vi "Site List to Site Numbers.vi"(0 "Site List":string) -> (4 "Site Numbers":i32[](array[numeric]), 6 "Sites":string[](array[string]))   [LabVIEW 2020]
uses:
  <vilib>/Utility/error.llb/whitespace.ctl
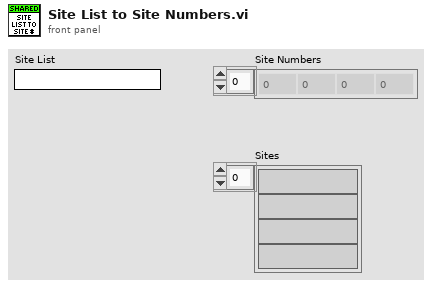
[diagram p1: front panel]
types:
  T1 = typedef "whitespace.ctl" = u16
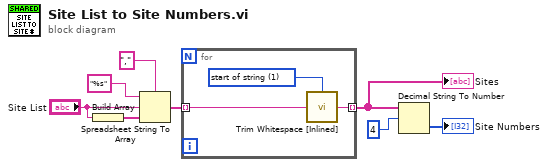
[diagram p0: block diagram]
diagram:
  n1 = Build Array("Site List") -> (w5:string[])
  n2 = Spreadsheet String To Array(delimiter (Tab)=",", format string="%s", spreadsheet string="Site List", array type (2D Dbl)=w5) -> (array=w4:string[])
  n3 = for {
    tunnel: w4 -> [w11] mode=indexing
    tunnel: [w9] -> w3 mode=indexing
    w10 = T1 1 items=["both", "start of string", "end of string"] ("location (both)")
    n4 = call "Trim Whitespace [Inlined].vi"("string"=w11, "location (both)"=w10) -> ("trimmed string"=w9:string)
  }
  "Sites" <- w3
  n5 = Decimal String To Number(string=w3, offset=4) -> (number=→"Site Numbers":i32[])  [unwired: 1 in, 1 out]
